vi "Build DS OpModes.vi"(6 "utility names":string[](array[string]), 9 "tele names":string[](array[string])=["TeleOp"], 11 "auto names":string[](array[string])=["Auto"]) -> ()   [LabVIEW 2026, in "MrcLib.lvlib"]
doc: "Simple way to update OpModes with named choices."
uses:
  MrcLib.lvlib
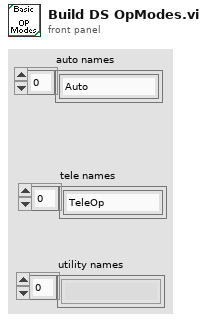
[diagram p1: front panel]
types:
  T1 = cluster{"hash":u64, "name":string, "group":string, "description":string, "text color":u32, "BG color":u32}
  T2 = cluster{"hash":u64, "name":string, "group":string, "description":string, "text color":u32, "BG color":u32}[]
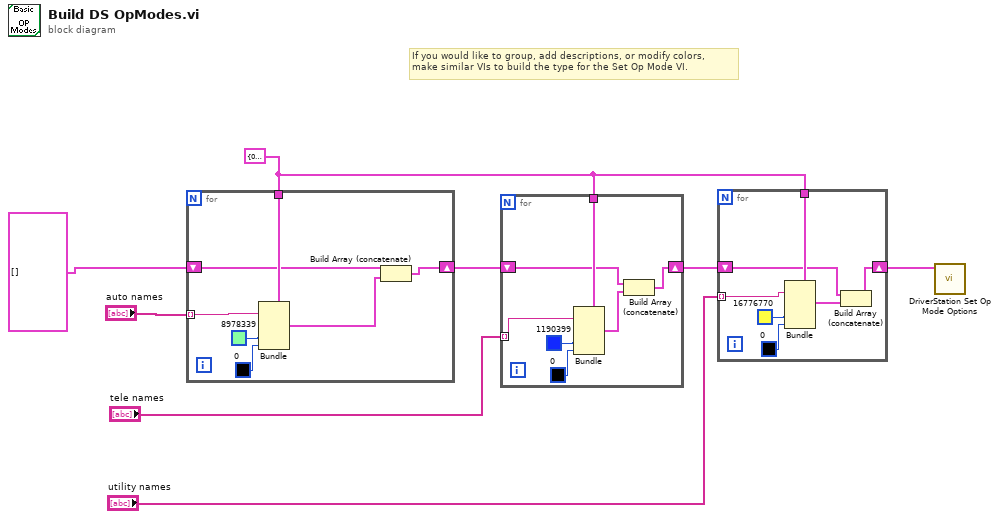
[diagram p0: block diagram]
diagram:
  w1 = T1 {"hash"=0, "name"="", "group"="", "description"="", "text color"=0, "BG color"=0} ("opModes out 2")
  # "If you would like to group, add descriptions, or modify colors,\nmake similar VIs to build the type for the Set Op Mode VI."
  n1 = for {
    tunnel: "auto names" -> [w14] mode=indexing
    shift-right: [w11] -> w5
    shift-left: T2 [] ("OpModes") -> [w10]
    tunnel: w1 -> [w15]
    n2 = Bundle(cluster=w15, "name"=w14, "text color"=u32 8978339, "BG color"=u32 0) -> (w9:T1)  [unwired: 3 in]
    n3 = Build Array (concatenate)(w10, w9) -> (w11:T2)
  }
  n4 = for {
    tunnel: "tele names" -> [w19] mode=indexing
    shift-right: [w18] -> w4
    shift-left: w5 -> [w16]
    tunnel: w1 -> [w20]
    n5 = Bundle(cluster=w20, "name"=w19, "text color"=u32 1190399, "BG color"=u32 0) -> (w17:T1)  [unwired: 3 in]
    n6 = Build Array (concatenate)(w16, w17) -> (w18:T2)
  }
  n7 = for {
    tunnel: "utility names" -> [w26] mode=indexing
    shift-right: [w23] -> w3
    shift-left: w4 -> [w25]
    tunnel: w1 -> [w27]
    n8 = Bundle(cluster=w27, "name"=w26, "text color"=u32 16776770, "BG color"=u32 0) -> (w24:T1)  [unwired: 3 in]
    n9 = Build Array (concatenate)(w25, w24) -> (w23:T2)
  }
  n10 = call "DriverStation Set Op Mode Options.vi"("opModes"=w3) -> ()  [unwired: 10 in, 1 out]
